vi "Receive String Data.vi"(8 "Error In":errorcluster, 9 "timeout ms (25000)":i32, 11 "TCP In":refnum<k5>) -> (0 "Error Out":errorcluster, 2 "String Data":string, 3 "TCP Out":refnum<k5>)   [LabVIEW 2012, in "OPI.lvclass"]
doc: "Receive string data prepend with big endian 4-byte size."
uses:
  OPI.lvclass
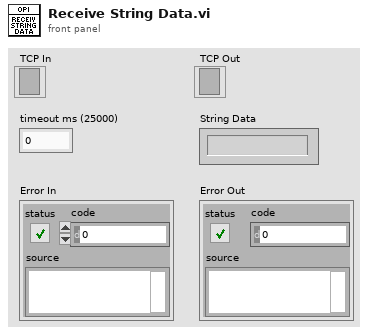
[diagram p1: front panel]
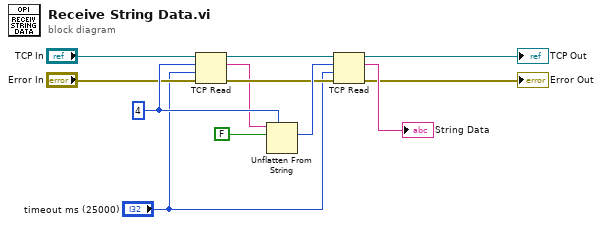
[diagram p0: block diagram]
diagram:
  w5 = 4 ("bytes to read")
  n1 = TCP Read(connection ID="TCP In", bytes to read=w5, error in (no error)="Error In", 9:"timeout ms (25000)") -> (connection ID out=w7:refnum<k5>, data out=w4:string, error out=w8:errorcluster)  [unwired: 1 in]
  n2 = Unflatten From String(type=w5, binary string=w4, data includes array or string size? (T)=FALSE) -> (value=w9:i32)  [unwired: 2 in, 2 out]
  n3 = TCP Read(connection ID=w7, bytes to read=w9, error in (no error)=w8, 9:"timeout ms (25000)") -> (connection ID out=→"TCP Out":refnum<k5>, data out=→"String Data":string, error out=→"Error Out":errorcluster)  [unwired: 1 in]
